vi "RenameReadEvents.vi"(1 "Read":refnum<user-event>[](array[refnum])) -> (0 "Read":refnum<user-event>[](array[refnum]))   [LabVIEW 2016, in "DAQ_Manager.lvclass"]
uses:
  DAQ_Manager.lvclass
  DAQ/Typedefs/PublicEvents--DAQ.Read.ctl
  DAQ/DAQ.lvclass
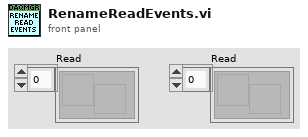
[diagram p1: front panel]
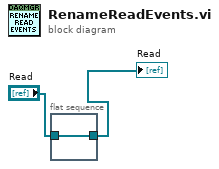
[diagram p0: block diagram]
diagram:
  n1 = flat-sequence {
    tunnel: [w3] -> w1
    tunnel: "Read" -> [w3]
    frame #0 {
    }
  }
  "Read" <- w1
